vi "Write Message[ ].vi"(8 "error in (no error)":errorcluster, 10 "Message[ ]":T1[](array[typedef]), 11 "Telegram Class in":refnum<class "Telegram Class.lvclass">) -> (0 "error out":errorcluster, 3 "Telegram Class out":refnum<class "Telegram Class.lvclass">)   [LabVIEW 2015, in "Telegram Library.lvlib" / "Telegram Class.lvclass"]
doc: "Created IvanLis by LabVIEW Portal\nProfile: http://labviewportal.org/memberlist.php?mode=viewprofile&u=987\neMail: IvanLisanov@gMail.com\nTelegram: https://t.me/IvanLis"
uses:
  Telegram Class.lvclass
  TypeDef/Message.ctl
  Telegram Class.lvclass/Telegram Class.ctl
  Telegram Library.lvlib
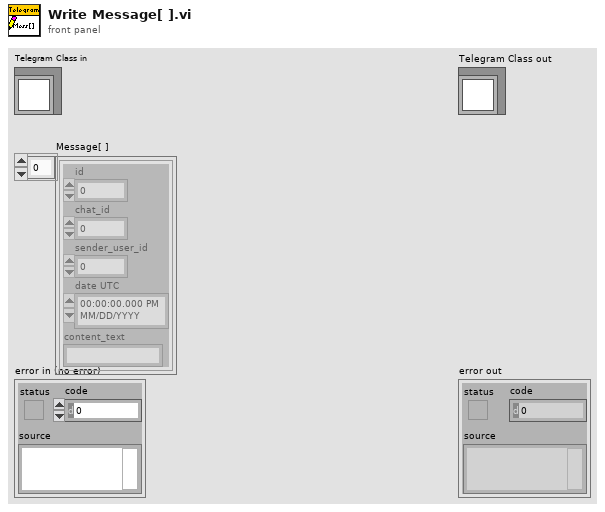
[diagram p1: front panel]
types:
  T1 = typedef "Telegram Library.lvlib/Message.ctl" = cluster{"id":i64, "chat_id":i64, "sender_user_id":i64, "date UTC":timestamp, "content_text":string}
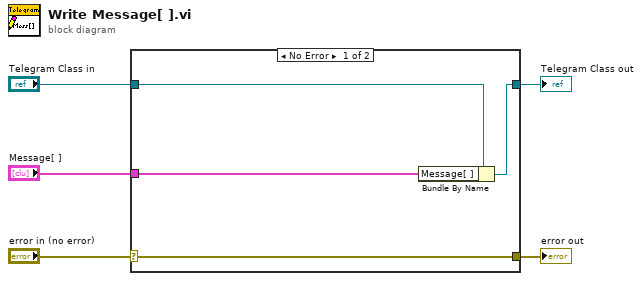
[diagram p0: block diagram]
diagram:
  n1 = case shown="No Error" "error in (no error)" {
    selector: "error in (no error)" -> [w9 w10]
    tunnel: [w9 w10] -> w4
    tunnel: [w7 w11] -> w2
    tunnel: "Telegram Class in" -> [w8 w11]
    tunnel: "Message[ ]" -> [w6 _]
    frame No Error {
      n2 = Bundle By Name(cluster=w8, "Message[ ]"=w6) -> (w7:refnum<class "Telegram Class.lvclass">)
    }
    frame Error {
    }
  }
  "error out" <- w4
  "Telegram Class out" <- w2
